vi "client.vi"() -> ()   [LabVIEW 2020]
panel:
  in  "module path":path
  out "return value":dbl[](array[numeric])
  in  "stop":bool
  out "error out":errorcluster
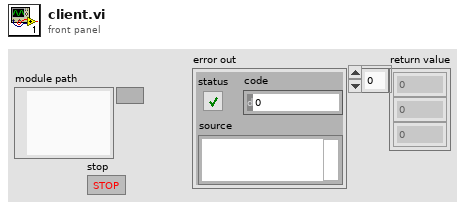
[diagram p1: front panel]
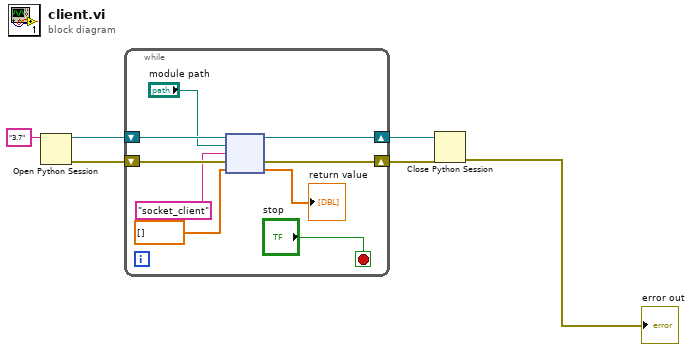
[diagram p0: block diagram]
diagram:
  n1 = Open Python Session(python version="3.7" ("Python version")) -> (session out=w6:refnum<k35>, error out=w5:errorcluster)  [unwired: 2 in]
  n2 = while {
    shift-right: [w13] -> w4
    shift-left: w6 -> [w15]
    shift-right: [w12] -> w3
    shift-left: w5 -> [w14]
    stop <- "stop" stop-if-true
    n3 = node(w15, "module path", "socket_client" ("function name"), w14, dbl[] []) -> (w13:refnum<k35>, w12:errorcluster, →"return value":dbl[])  [unwired: 2 out]
  }
  n4 = Close Python Session(session in=w4, error in=w3) -> (11:→"error out":errorcluster)
